vi "MGI Tree Rows from Delimited String Array.vi"(8 "Use Child Only? (False)":bool, 9 "Default Symbol":i32, 10 "Delimiter":string="\\", 11 "Items (Delimited)":string[][](array[string])) -> (2 "Parent Tag Added[]":string[](array[string]), 3 "Item to Add[]":T1(array[cluster]))   [LabVIEW 2016]
doc: "Convert the array of delimited strings stored in the first column of the specified array to Tree Rows. The remaining columns are used as text for each tree row.\n\nAuthored by Shawn D. Walpole\nsupport@mooregoodideas.com\nwww.mooregoodideas.com\n\nCopyright (c) 2010, Moore Good Ideas, Inc.\n\nAll rights reserved.\n\nRedistribution and use in source and binary forms, with or without modification, are permitted provided that the following conditions are met:\n\n * Redistributions of source code must retain the above copyright notice, this list of conditions and the following disclaimer.\n * Redistributions in binary form must reproduce the above copyright notice, this list of conditions and the following disclaimer in the documentation and/or other materials provided with the distribution.\n * Neither the name of Moore Good Ideas, Inc. nor the names of its contributors may be used to endorse or promote products derived from this software without specific prior written permission.\n\nTHIS SOFTWARE IS PROVIDED BY THE COPYRIGHT HOLDERS AND CONTRIBUTORS \"AS IS\" AND ANY EXPRESS OR IMPLIED WARRANTIES, INCLUDING, BUT NOT LIMITED TO, THE IMPLIED WARRANTIES OF MERCHANTABILITY AND FITNESS FOR A PARTICULAR PURPOSE ARE DISCLAIMED. IN NO EVENT SHALL THE COPYRIGHT OWNER OR CONTRIBUTORS BE LIABLE FOR ANY DIRECT, INDIRECT, INCIDENTAL, SPECIAL, EXEMPLARY, OR CONSEQUENTIAL DAMAGES (INCLUDING, BUT NOT LIMITED TO, PROCUREMENT OF SUBSTITUTE GOODS OR SERVICES; LOSS OF USE, DATA, OR PROFITS; OR BUSINESS INTERRUPTION) HOWEVER CAUSED AND ON ANY THEORY OF LIABILITY, WHETHER IN CONTRACT, STRICT LIABILITY, OR TORT (INCLUDING NEGLIGENCE OR OTHERWISE) ARISING IN ANY WAY OUT OF THE USE OF THIS SOFTWARE, EVEN IF ADVISED OF THE POSSIBILITY OF SUCH DAMAGE."
panel:
  out "Index":i32
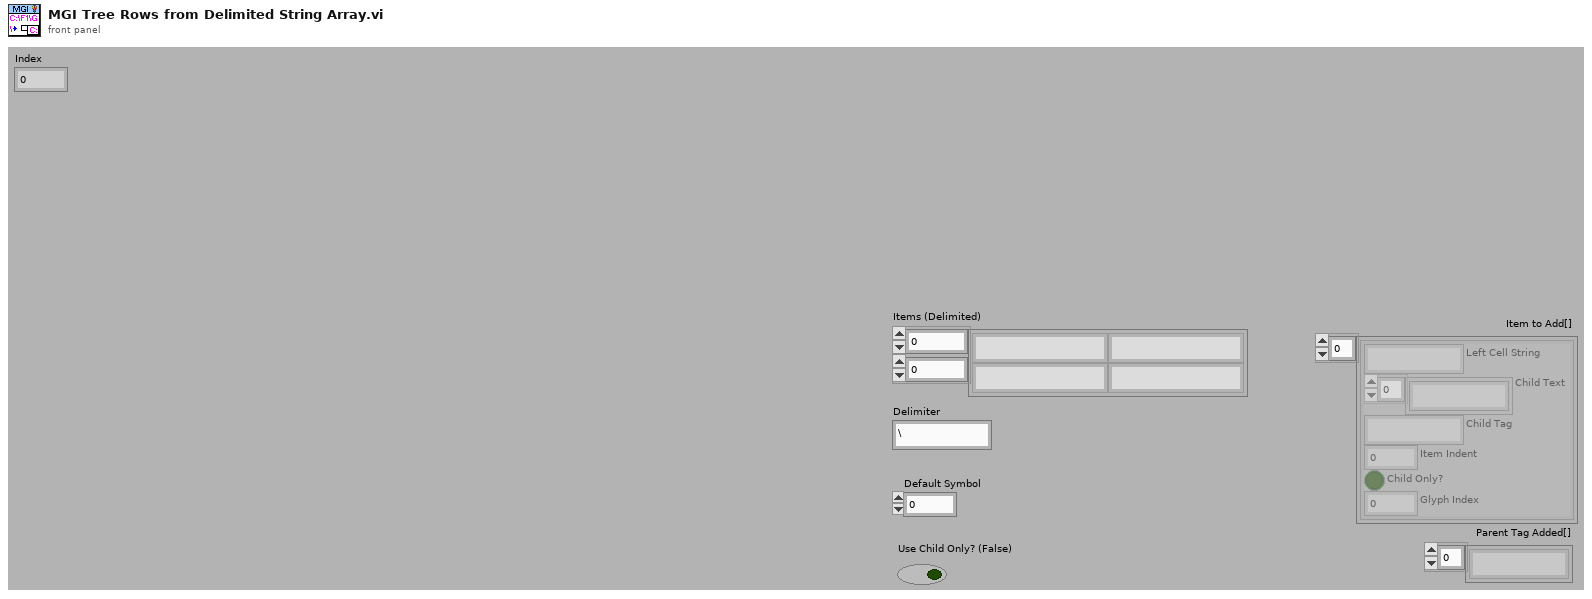
[diagram p1: front panel]
types:
  T1 = cluster{"Left Cell String":string, "Child Text":string[], "Child Tag":string, "Item Indent":i32, "Child Only?":bool, "Glyph Index":i32}[]
  T2 = cluster{"Left Cell String":string, "Child Text":string[], "Child Tag":string, "Item Indent":i32, "Child Only?":bool, "Glyph Index":i32}
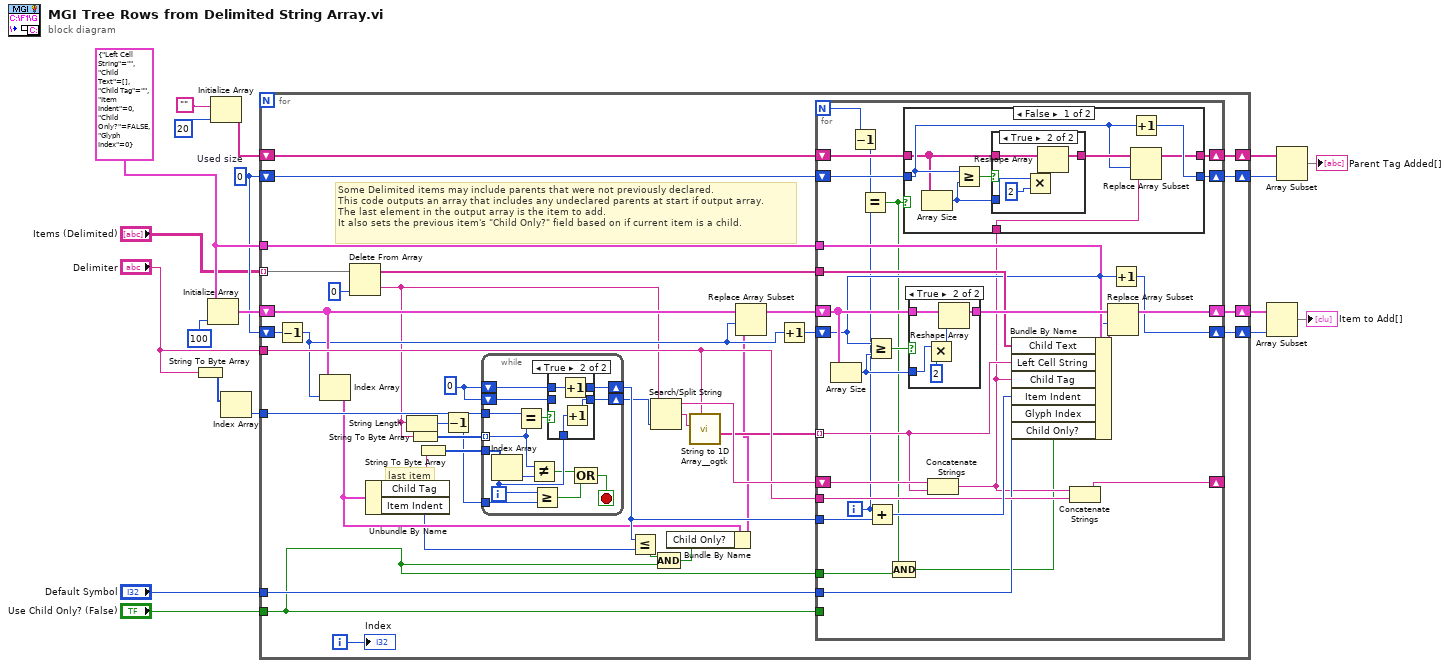
[diagram p0: block diagram]
diagram:
  w2 = 0  # Used size
  w8 = T2 {"Left Cell String"="", "Child Text"=[], "Child Tag"="", "Item Indent"=0, "Child Only?"=FALSE, "Glyph Index"=0} ("Item")
  n1 = String To Byte Array(string="Delimiter") -> (unsigned byte array=w18:u8[])
  n2 = Initialize Array(w8, 100 ("dimension size")) -> (w15:T1)
  n3 = Initialize Array("", 20 ("dimension size")) -> (w14:string[])
  n4 = Index Array(array=w18) -> (element=w19:u8)  [unwired: 1 in]
  n5 = for {
    shift-right: [w54] -> w17
    shift-left: w2 -> [w43]
    shift-right: [w55] -> w16
    shift-left: w15 -> [w44]
    tunnel: "Items (Delimited)" -> [w56] mode=indexing
    tunnel: "Delimiter" -> [w48]
    tunnel: w8 -> [w52]
    tunnel: w19 -> [w50]
    tunnel: "Default Symbol" -> [w45]
    tunnel: "Use Child Only? (False)" -> [w39]
    shift-right: [w36] -> w11
    shift-left: w14 -> [w38]
    shift-right: [w35] -> w10
    shift-left: w2 -> [w37]
    i -> [w51]
    w29 = 0
    # "last item"
    # "Some Delimited items may include parents that were not previously declared.\nThis code outputs an array that includes any undeclared parents at start if output array.\nThe last element in the output array is the item to add.\nIt also sets the previous item's \"Child Only?\" field based on if current item is a child."
    n6 = Decrement(x=w43) -> (x-1=w42:i32)
    n7 = Index Array(array=w44, index=w42) -> (element=w27:T2)
    n8 = Delete From Array(array=w56, index=0) -> (deleted portion=w22:string, array with subset deleted=w53:string[])  [unwired: 1 in]
    n9 = Unbundle By Name(w27) -> ("Child Tag"=w33:string, "Item Indent"=w24:i32)
    n10 = String Length(string=w22) -> (length=w21:i32)
    n11 = String To Byte Array(string=w22) -> (unsigned byte array=w32:u8[])
    n12 = String To Byte Array(string=w33) -> (unsigned byte array=w31:u8[])
    n13 = Decrement(x=w21) -> (x-1=w20:i32)
    n14 = while {
      shift-right: [w64] -> w46
      shift-left: w29 -> [w65]
      tunnel: w32 -> [w68] mode=indexing
      tunnel: w31 -> [w70]
      tunnel: w50 -> [w67]
      shift-right: [w63] -> w28
      shift-left: w29 -> [w62]
      tunnel: w20 -> [w60]
      i -> [w59]
      stop <- w61 stop-if-true
      n15 = Index Array(array=w70, index=w59) -> (element=w69:u8)
      n16 = Equal?(x=w67, y=w68) -> (x = y?=w66:bool)
      n17 = Not Equal?(x=w68, y=w69) -> (x != y?=w57:bool)
      n18 = Greater Or Equal?(x=w59, y=w60) -> (x >= y?=w58:bool)
      n19 = case shown="True" w66 {
        tunnel: w65 -> [w72 w76]
        tunnel: w62 -> [w71 _]
        tunnel: [w72 w75] -> w64
        tunnel: w59 -> [_ w74]
        tunnel: [w71 w73] -> w63
        frame False {
        }
        frame True {
          n20 = Increment(x=w76) -> (x+1=w75:i32)
          n21 = Increment(x=w74) -> (x+1=w73:i32)
        }
      }
      n22 = Compound Arithmetic op=OR(w57, w58) -> (w61:bool)
    }
    n23 = Less Or Equal?(x=w46, y=w24) -> (x <= y?=w23:bool)
    n24 = Search/Split String(string=w22, offset (0)=w28) -> (substring before match=w49:string, match + rest of string=w30:string)  [unwired: 1 in, 1 out]
    n25 = Compound Arithmetic op=AND(w23, w39) -> (w25:bool)
    n26 = Bundle By Name(cluster=w27, "Child Only?"=w25) -> (w26:T2)
    n27 = call <userlib>:"String to 1D Array__ogtk.vi"("delimiter (Tab)"=w48, "string"=w30) -> ("Array of Strings"=w47:string[])  [unwired: 1 in, 8 out]
    n28 = Replace Array Subset(array=w44, new element=w26, index=w42) -> (w41:T1)
    n29 = Increment(x=w42) -> (x+1=w40:i32)
    n30 = for {
      N -> [w81]
      shift-right: [w101] -> w55
      shift-left: w41 -> [w104]
      shift-right: [w89] -> w54
      shift-left: w40 -> [w90]
      tunnel: w53 -> [w97]
      tunnel: w52 -> [w99]
      shift-right: [w93] -> _
      shift-left: w49 -> [w96]
      tunnel: w48 -> [w94]
      tunnel: w46 -> [w92]
      tunnel: w47 -> [w91] mode=indexing
      tunnel: w45 -> [w88]
      tunnel: w39 -> [_]
      tunnel: w39 -> [w78]
      shift-right: [w85] -> w36
      shift-left: w38 -> [w84]
      shift-right: [w86] -> w35
      shift-left: w37 -> [w87]
      i -> [w82]
      n31 = Array Size(array=w104) -> (size(s)=w102:i32)
      n32 = Decrement(x=w81) -> (x-1=w80:i32)
      n33 = Equal?(x=w80, y=w82) -> (x = y?=w79:bool)
      n34 = Greater Or Equal?(x=w90, y=w102) -> (x >= y?=w103:bool)
      n35 = Add(x=w82, y=w92) -> (x+y=w95:i32)
      n36 = Compound Arithmetic op=AND(w79, w78) -> (w77:bool)
      n37 = case shown="True" w103 {
        tunnel: w104 -> [w121 w124]
        tunnel: [w121 w126] -> w100
        tunnel: w102 -> [_ w122]
        frame False {
        }
        frame True {
          n38 = Multiply(x=w122, y=2) -> (x*y=w125:i32)
          n39 = Reshape Array(w124, w125) -> (w126:T1)
        }
      }
      n40 = Concatenate Strings(w96, w91) -> (w83:string)
      n41 = case shown="False" w79 {
        tunnel: w87 -> [w110 w119]
        tunnel: [w109 w119] -> w86
        tunnel: [w108 w120] -> w85
        tunnel: w84 -> [w106 w120]
        tunnel: w83 -> [w105 _]
        frame False {
          n42 = Array Size(array=w106) -> (size(s)=w112:i32)
          n43 = Greater Or Equal?(x=w110, y=w112) -> (x >= y?=w107:bool)
          n44 = case shown="True" w107 {
            tunnel: w106 -> [w113 w116]
            tunnel: [w113 w118] -> w111
            tunnel: w112 -> [_ w114]
            frame False {
            }
            frame True {
              n45 = Multiply(x=w114, y=2) -> (x*y=w117:i32)
              n46 = Reshape Array(w116, w117) -> (w118:string[])
            }
          }
          n47 = Increment(x=w110) -> (x+1=w109:i32)
          n48 = Replace Array Subset(array=w111, new element=w105, index=w110) -> (w108:string[])
        }
        frame True {
        }
      }
      n49 = Bundle By Name(cluster=w99, "Child Text"=w97, "Left Cell String"=w91, "Child Tag"=w83, "Item Indent"=w95, "Glyph Index"=w88, "Child Only?"=w77) -> (w98:T2)
      n50 = Concatenate Strings(w83, w94) -> (w93:string)
      n51 = Replace Array Subset(array=w100, new element=w98, index=w90) -> (w101:T1)
      n52 = Increment(x=w90) -> (x+1=w89:i32)
    }
    "Index" <- w51
  }
  n53 = Array Subset(array=w16, length=w17) -> (→"Item to Add[]":T1)  [unwired: 1 in]
  n54 = Array Subset(array=w11, length=w10) -> (→"Parent Tag Added[]":string[])  [unwired: 1 in]
